vi "GEA2 Read Message.vi"(0 "GEA2 Reference In":refnum<k24>, 5 "Expected Command":string=".*", 7 "Expected Data":string=".*", 9 "Timeout":u32=500, 11 "Error In":errorcluster) -> (4 "GEA2 Reference Out":refnum<k24>, 6 "Raw Data Out":string, 8 "Coverted Data Out":T1 {"CRC" format="%04x"; "Length" format="%02x"; "Command" format="%02x"; "Destination" format="%02x"; "Source" format="%02x"}, 15 "Error Out":errorcluster)   [LabVIEW 2014, in "GEA2_Toolkit.lvlib"]
doc: "This VI accepts an event registration input. The input event is generated every time a message is present on the GEA2 bus. When an event is detected the event structure exectures and the output of this VI contains source and destination address as well as the command and data."
uses:
  library/GEA2_Toolkit.lvlib
  C:/Automation/DLLs/PC Tools .NET/GeaCommunication.dll
  Automation/DLLs/PC Tools .NET/GeaCommunication.dll
  type defs/Data Out.ctl
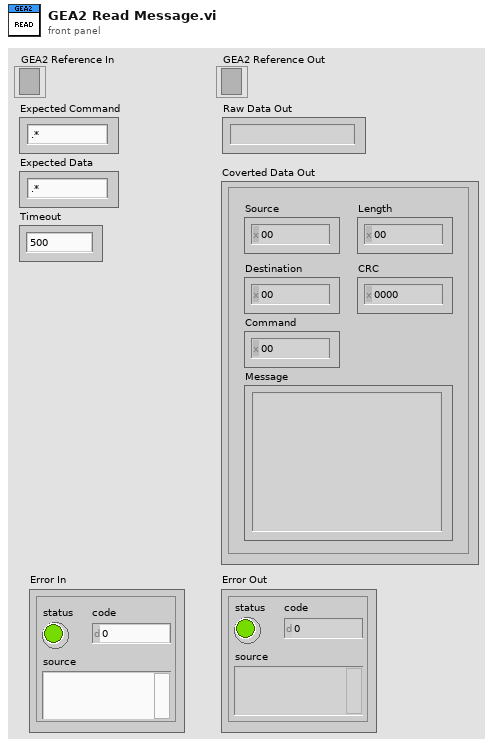
[diagram p1: front panel]
types:
  T1 = typedef "GEA2_Toolkit.lvlib/Data Out.ctl" = cluster{"Source":u8, "Destination":u8, "Command":u8, "Length":u8, "CRC":u16, "Message":string}
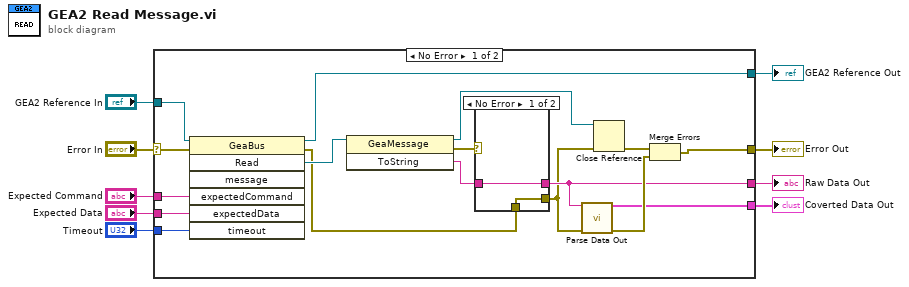
[diagram p0: block diagram]
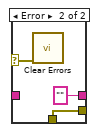
[diagram p2: hidden frame]
diagram:
  n1 = case shown="No Error" "Error In" {
    selector: "Error In" -> [w21 w32]
    tunnel: "GEA2 Reference In" -> [w25 w33]
    tunnel: [w20 w33] -> w6
    tunnel: [w14 w32] -> w8
    tunnel: "Expected Command" -> [w24 _]
    tunnel: "Expected Data" -> [w23 _]
    tunnel: "Timeout" -> [w22 _]
    tunnel: [w13 _] -> w2
    tunnel: [w12 _] -> w1
    frame No Error {
      n2 = invoke class="GeaBus" method="Read"(reference=w25, error in=w21, "expectedCommand"=w24, "expectedData"=w23, "timeout"=w22) -> (reference out=w20:refnum<k24>, error out=w10:errorcluster, "Read"=w26:refnum<k24>)  [unwired: 2 in, 4 out]
      n3 = invoke class="GeaMessage" method="ToString"(reference=w26) -> (reference out=w17:refnum<k24>, error out=w18:errorcluster, "ToString"=w19:string)  [unwired: 2 in]
      n4 = case shown="No Error" w18 {
        selector: w18 -> [_ w30]
        tunnel: w19 -> [w28 _]
        tunnel: [w28 "" ("ToString")] -> w13
        tunnel: [w27 w29] -> w11
        tunnel: w10 -> [w27 w29]
        frame No Error {
        }
        frame Error {
          n5 = call <vilib>:"Clear Errors.vi"("error in (no error)"=w30) -> ()  [unwired: 5 in, 2 out]
        }
      }
      n6 = call "Parse Data Out.vi"("Raw Data In"=w13, "Error In"=w11) -> ("Data Out"=w12:T1, "Error Out"=w15:errorcluster)  [unwired: 12 in]
      n7 = Close Reference(reference=w17, error in (no error)=w11) -> (error out=w16:errorcluster)
      n8 = Merge Errors(w16, w15) -> (w14:errorcluster)
    }
    frame Error {
    }
  }
  "Error Out" <- w8
  "GEA2 Reference Out" <- w6
  "Raw Data Out" <- w2
  "Coverted Data Out" <- w1
